vi "svl_Log View for Energy Level (array).vi"(7 "channel info":T1={"sensor sensitivity"=1000.0, "engineering units"=1, "dB reference"=1.0, "custom label"="EU", "weighting filter"=0, "pregain"=0.0} {"pregain" format="%.2f"; "weighting filter" items=["Linear", "A-weighting", "B-weighting", "C-weighting", "ITU-R 468-4", "Dolby", "CCITT", "C-message", "Wb", "Wc", "Wd", "We", "Wf", "Wh", "Wj", "Wk", "Wm", "AES17 20 kHz lowpass", "AES17 40 kHz lowpass", "AES17 20 kHz highpass", "AES17 40 kHz highpass"]; "dB reference" format="%^.1e"; "engineering units" items=["custom..."=0, "V"=1, "A"=21, "C"=30, "pC"=31, "s"=32, "-"=29, "Pa"=2, "N"=20, "g"=3, "m/s^2"=4, "m/s"=5, "m"=6, "mm/s"=12, "mm"=13, "micron/s"=14, "micron"=15, "in/s^2"=7, "in/s"=8, "in"=9, "mil/s"=10, "mil"=11, "rad/s^2"=16, "rad/s"=17, "rad"=18, "deg/s^2"=26, "deg/s"=27, "deg"=28, "RPM"=22, "cycle/s^2"=23, "Hz"=24, "cycle"=25, "strain"=19]; "sensor sensitivity" format="%#_5f"}, 8 "error in (no error)":errorcluster, 9 "view mode":enum16{"Power", "Amplitude"}(ring), 10 "dB On (T)":bool=TRUE, 11 "scaled signal":dbl[](array[numeric])) -> (0 "error out":errorcluster, 2 "unit label":string, 3 "log view scaled signal":dbl[](array[numeric]))   [LabVIEW 2017]
uses:
  <vilib>/addons/_NISVFA/_Shared subVIs/Controls/svc_Channel Info.ctl
  <vilib>/addons/_NISVFA/_Shared subVIs/Controls/svc_Engineering Units Text Ring.ctl
  <vilib>/addons/_NISVFA/_Shared subVIs/Controls/svc_Weighting Filter Text Ring.ctl
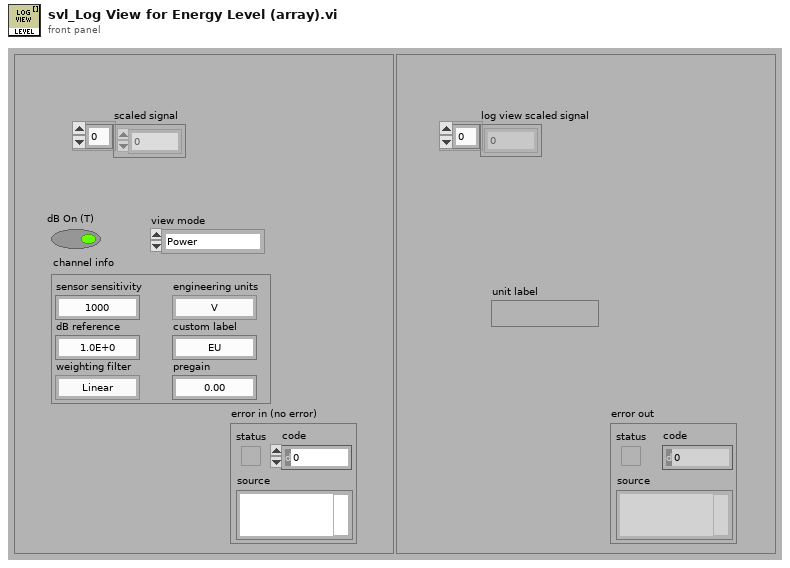
[diagram p1: front panel]
types:
  T1 = typedef "svc_Channel Info.ctl" = cluster{"sensor sensitivity":dbl, "engineering units":T2, "dB reference":dbl, "custom label":string, "weighting filter":T3, "pregain":dbl}
  T2 = typedef "svc_Engineering Units Text Ring.ctl" = u16
  T3 = typedef "svc_Weighting Filter Text Ring.ctl" = u16
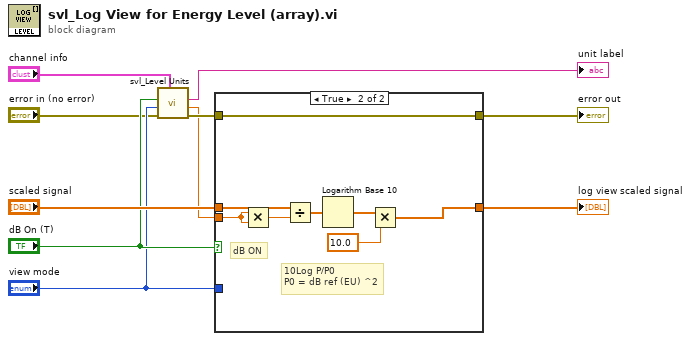
[diagram p0: block diagram]
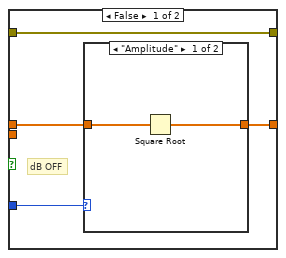
[diagram p2: hidden frame]
diagram:
  n1 = call <vilib>:"svl_Level Units.vi"("channel info"="channel info", "error in (no error)"="error in (no error)", "view mode"="view mode", "dB On (T)"="dB On (T)") -> ("error out"=w4:errorcluster, "dB reference [EU]"=w3:dbl, "unit label"=→"unit label":string)  [unwired: 5 in]
  n2 = case shown="True" "dB On (T)" {
    tunnel: [w14 w20] -> w8
    tunnel: w4 -> [w13 w25]
    tunnel: [w13 w25] -> w10
    tunnel: "scaled signal" -> [w11 w21]
    tunnel: "view mode" -> [w12 _]
    tunnel: w3 -> [_ w19]
    frame False {
      # "dB OFF"
      n3 = case shown="\"Amplitude\"" w12 {
        tunnel: [w15 w17] -> w14
        tunnel: w11 -> [w16 w17]
        frame "Amplitude" {
          n4 = Square Root(x=w16) -> (sqrt(x)=w15:dbl[])
        }
        frame "Power", Default {
        }
      }
    }
    frame True {
      # "10Log P/P0\nP0 = dB ref (EU) ^2"
      # "dB ON"
      n5 = Multiply(x=w19, y=w19) -> (x*y=w18:dbl)
      n6 = Divide(x=w21, y=w18) -> (x/y=w22:dbl[])
      n7 = Logarithm Base 10(1:w22) -> (0:w23:dbl[])
      n8 = Multiply(x=w23, y=10.0) -> (x*y=w20:dbl[])
    }
  }
  "log view scaled signal" <- w8
  "error out" <- w10
